vi "Auto_Routine_BlueStraightThreePieceLeftNoteTRAJ.vi"(8 "error in (no error)":errorcluster) -> (0 "error out":errorcluster)   [LabVIEW 2023]
uses:
  Trajectory/TrajectoryGlobals.vi
  Arm2/ArmGetSetpointEnum.ctl
  <vilib>/Rock Robotics/WPI/ThirdParty/JAS_Junk/TrajLib/Trajectory_Library.lvlib
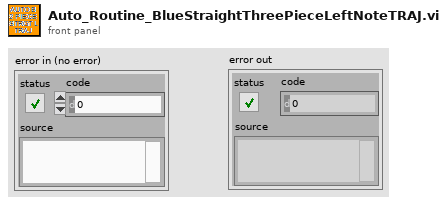
[diagram p1: front panel]
types:
  T1 = typedef "Trajectory_Library.lvlib/TRAJECTORY.ctl" = cluster{"TotalTImeSecs":dbl, "States":T2[]}
  T2 = typedef "Trajectory_Library.lvlib/TRAJ_STATE.ctl" = cluster{"TimeSeconds":dbl, "Velocity":dbl, "Acceleration":dbl, "POSE":T3, "Curvature":dbl}
  T3 = typedef "Trajectory_Library.lvlib/POSE2D.ctl" = cluster{"TRANSLATION":T4, "ROTATION":T5}
  T4 = typedef "Trajectory_Library.lvlib/TRANSLATION2D.ctl" = cluster{"X":dbl, "Y":dbl}
  T5 = typedef "Trajectory_Library.lvlib/ROTATION2D.ctl" = cluster{"VALUE":dbl, "COS":dbl, "SIN":dbl}
  T6 = typedef "ArmGetSetpointEnum.ctl" = enum16{"ArmFloorPickup", "ArmAmpDeposit", "ArmSpeakerShoot", "ArmStartPosition", "ArmRestPosition", "ArmSourceIntake", "ArmAwayShoot"}
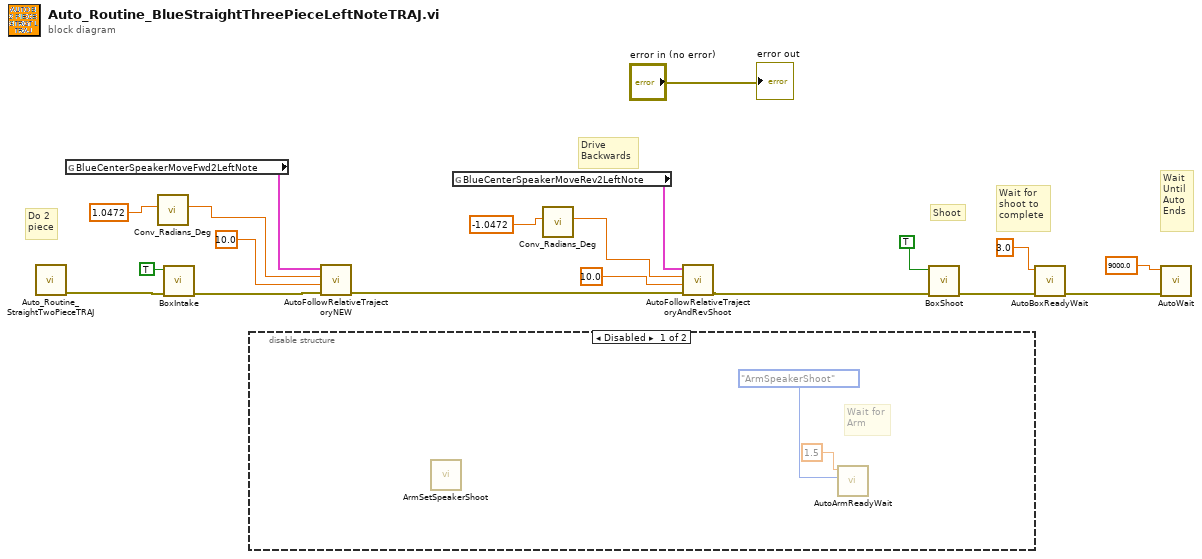
[diagram p0: block diagram]
diagram:
  # "Do 2 \npiece"
  # "Wait for\nshoot to\ncomplete"
  # "Shoot"
  # "Drive\nBackwards"
  # "Wait\nUntil\nAuto \nEnds"
  n1 = call "Auto_Routine_StraightTwoPieceTRAJ.vi"() -> ("error out"=w4:errorcluster)  [unwired: 11 in]
  n2 = global read "TrajectoryGlobals.vi" "BlueCenterSpeakerMoveFwd2LeftNote"() -> (w18:T1)
  n3 = call <vilib>:"Conv_Radians_Deg.vi"("Radians"=1.0472) -> ("Degrees"=w16:dbl)  [unwired: 10 in]
  n4 = call "BoxIntake.vi"("error in (no error)"=w4, "Box intake"=TRUE) -> ("error out"=w5:errorcluster)  [unwired: 9 in]
  n5 = disable-structure shown="Disabled" {
    frame Disabled {
      # "Wait for\nArm"
      n6 = call "ArmSetSpeakerShoot.vi"() -> ()  [unwired: 11 in, 1 out]
      n7 = call "AutoArmReadyWait.vi"("ArmSetpoints"=ArmGetSetpointEnum."ArmSpeakerShoot", "TimeOut (s)"=1.5) -> ("error out"=w21:errorcluster, "error in (no error)"=w20:errorcluster)  [unwired: 8 in]
    }
    frame Enabled {
    }
  }
  n8 = call "AutoFollowRelativeTrajectoryNEW.vi"("error in (no error)"=w5, "TimeOut (s)"=10.0, "End Orientation"=w16, "Trajectory"=w18) -> ("error out"=w2:errorcluster)  [unwired: 7 in]
  n9 = global read "TrajectoryGlobals.vi" "BlueCenterSpeakerMoveRev2LeftNote"() -> (w10:T1)
  n10 = call <vilib>:"Conv_Radians_Deg.vi"("Radians"=-1.0472) -> ("Degrees"=w8:dbl)  [unwired: 10 in]
  n11 = call "AutoFollowRelativeTrajectoryAndRevShoot.vi"("error in (no error)"=w2, "TimeOut (s)"=10.0, "End Orientation"=w8, "Trajectory"=w10) -> ("error out"=w1:errorcluster)  [unwired: 7 in]
  n12 = call "BoxShoot.vi"("error in (no error)"=w1, "Box shoot"=TRUE) -> ("error out"=w13:errorcluster)  [unwired: 9 in]
  n13 = call "AutoBoxReadyWait.vi"("error in (no error)"=w13, "TimeOut (s)"=3.0) -> ("error out"=w11:errorcluster)  [unwired: 9 in]
  n14 = call "AutoWait.vi"("error in (no error)"=w11, "TimeOut (s)"=9000.0) -> ()  [unwired: 9 in, 1 out]
  "error out" <- "error in (no error)"
